vi "OverlayTest.vi"() -> ()   [LabVIEW 2015]
panel:
  in  "Listbox":i32(listbox)
  out "Center":dbl
  in  "BullseyeLocation":T1={"X Center"=364, "Y Center"=60, "Height"=92, "Width"=57}
  out "Image":T2(plugin-control)
  in  "index":i32
  out "Object Info.Bounding Box":T3={"X Left"=341, "Y Top"=61, "X Right"=396, "Y Bottom"=95}
  in  "End Point 2":cluster{"X":i32, "Y":i32}={"X"=450, "Y"=320}
  in  "Start Point 2":cluster{"X":i32, "Y":i32}={"X"=600, "Y"=480}
  in  "End Point":cluster{"X":i32, "Y":i32}={"X"=160, "Y"=320}
  in  "Start Point":cluster{"X":i32, "Y":i32}={"X"=15, "Y"=480}
  in  "stop":bool
  out "Masked":T2(plugin-control)
  out "Box Center":dbl=367.3384704589844
  in  "BallPresent":T4={"X Offset"=140, "Y Offset"=0, "Diameter"=20}
  in  "FixedMarkers":dbl[](array[numeric])
  in  "Value":dbl(slide)=1.0 scale=0.0..1.0
  in  "LinearLocation":T5={"X Offset"=10, "Y Offset"=170, "Height"=300, "Width"=10}
  in  "Values":dbl[](array[numeric])=[5000.0, 5129.0, 6.2, 1568.0]
  in  "Headers":string[](array[string])=["RPM:  ", "RPMt: ", "Box Pos: ", "Blah: "]
  in  "Present?":bool
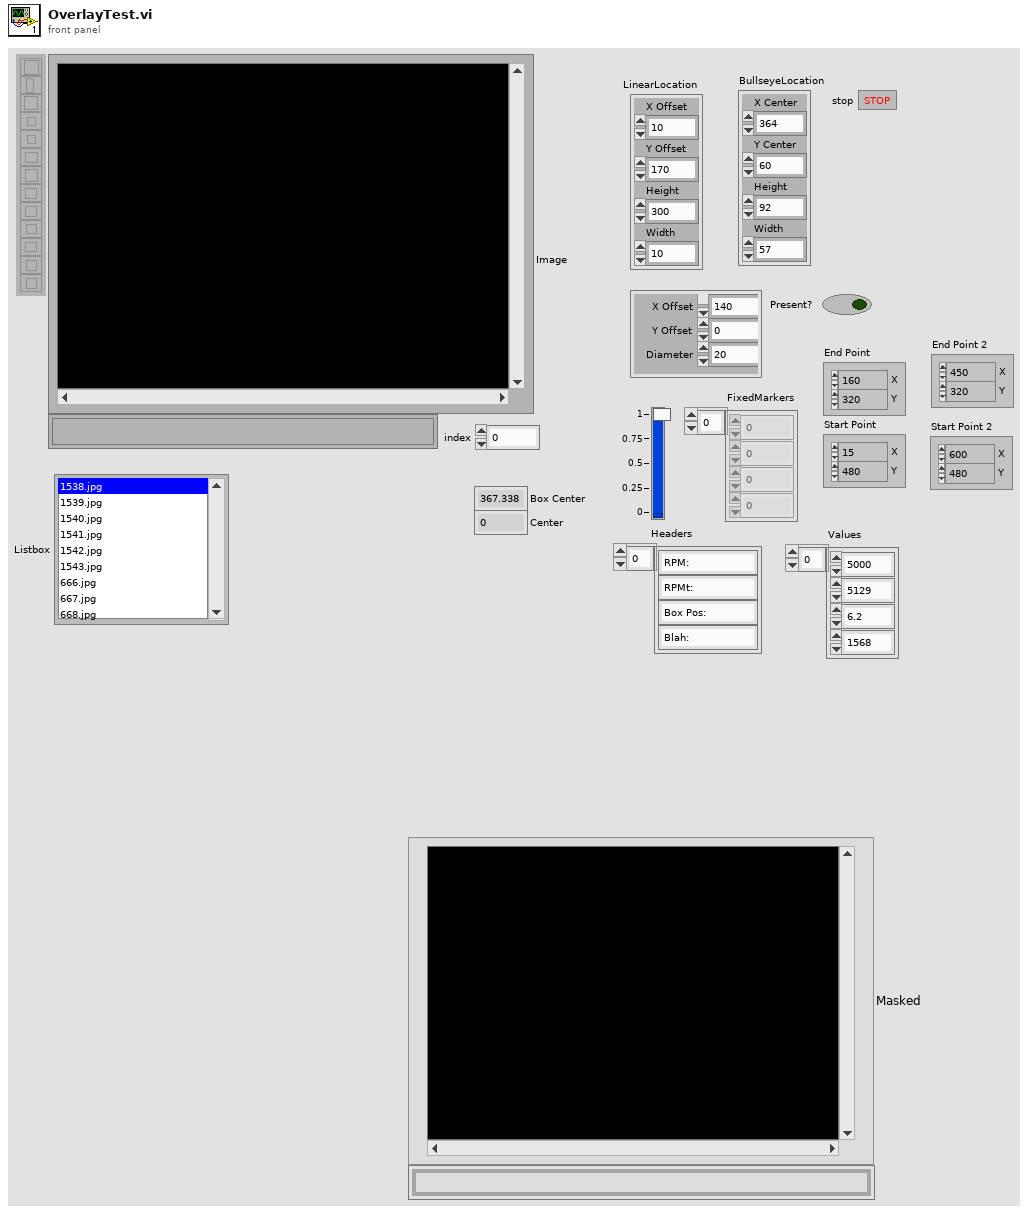
[diagram p1: front panel]
types:
  T1 = cluster{"X Center":i32, "Y Center":i32, "Height":i32, "Width":i32}
  T2 = typedef "IMAQ Image.ctl" = refnum<image>
  T3 = cluster{"X Left":i32, "Y Top":i32, "X Right":i32, "Y Bottom":i32}
  T4 = cluster{"X Offset":i32, "Y Offset":i32, "Diameter":i32}
  T5 = cluster{"X Offset":i32, "Y Offset":i32, "Height":i32, "Width":i32}
  T6 = typedef "Image Type" = u32
  T7 = cluster{"Area":sgl, "Object Info":cluster{"Object Center":cluster{"X":sgl, "Y":sgl}, "Bounding Box":cluster{"X Left":i32, "Y Top":i32, "X Right":i32, "Y Bottom":i32}, "Area":sgl, "Orientation":sgl, "Aspect Ratio":sgl, "Nb Holes":i32}}[]
  T8 = typedef "Scores.ctl" = cluster{"Bounding box":cluster{"left":dbl, "top":dbl, "right":dbl, "bottom":dbl}, "Aspect Ratio":dbl, "Area to CH":dbl, "X Mask":dbl, "Y Mask":dbl, "Moment":dbl, "Center":dbl}
  T9 = cluster{cluster{"Left":dbl, "Top":dbl, "Right":dbl, "Bottom":dbl}, "Scores":dbl[], cluster{"Long":dbl, "Short":dbl}}[]
  T10 = cluster{cluster{"Left":dbl, "Top":dbl, "Right":dbl, "Bottom":dbl}, "Scores":dbl[], cluster{"Long":dbl, "Short":dbl}}
  T11 = cluster{"Area":sgl, "Object Info":cluster{"Object Center":cluster{"X":sgl, "Y":sgl}, "Bounding Box":cluster{"X Left":i32, "Y Top":i32, "X Right":i32, "Y Bottom":i32}, "Area":sgl, "Orientation":sgl, "Aspect Ratio":sgl, "Nb Holes":i32}}
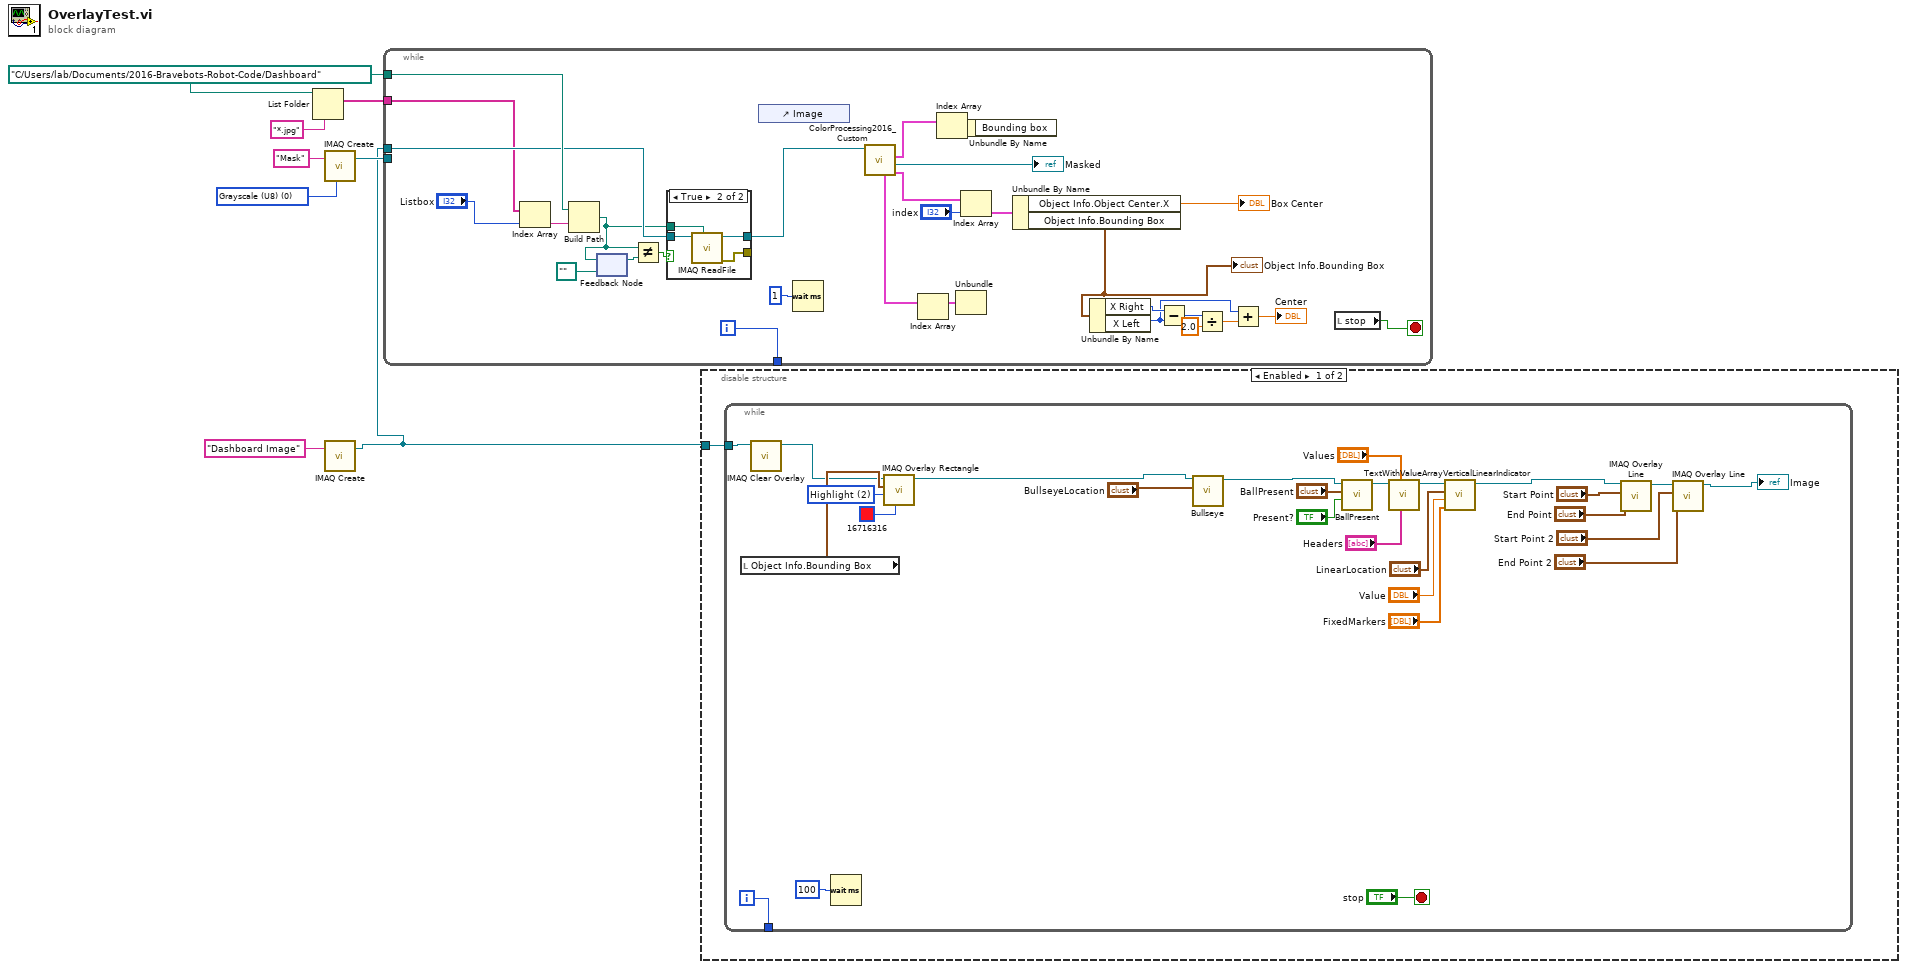
[diagram p0: block diagram]
diagram:
  w3 = path "C:/Users/lab/Documents/2016-Bravebots-Robot-Code/Dashboard" ("File Path")
  w7 = T6 0 items=["Grayscale (U8)", "Grayscale (I16)", "Grayscale (SGL)", "Complex (CSG)", "RGB (U32)", "HSL (U32)", "RGB (U64)", "Grayscale (U16)"] ("Image Type")
  n1 = List Folder(path=w3, pattern="*.jpg") -> (filenames=w2:string[])  [unwired: 2 in, 3 out]
  n2 = call "IMAQ Create"("Image Name"="Mask", "Image Type"=w7) -> ("New Image"=w5:T2)  [unwired: 2 in, 2 out]
  n3 = call "IMAQ Create"("Image Name"="Dashboard Image") -> ("New Image"=w1:T2)  [unwired: 3 in, 2 out]
  n4 = while {
    tunnel: w1 -> [w14]
    tunnel: w5 -> [_]
    tunnel: [w32] -> _
    tunnel: w3 -> [w18]
    tunnel: w2 -> [w12]
    i -> [w32]
    stop <- w31 stop-if-true
    n5 = Index Array(array=w12, index="Listbox") -> (element=w10:string)
    n6 = Build Path(base path=w18, name or relative path=w10) -> (appended path=w9:path)
    n7 = feedback #1(path "" ("appended path")) -> (w17:path)
    n8 = feedback-in #1(w9) -> ()
    n9 = Not Equal?(x=w9, y=w17) -> (x != y?=w15:bool)
    n10 = case shown="True" w15 {
      tunnel: [w38 w42] -> w13
      tunnel: [_ w41] -> _
      tunnel: w14 -> [w38 w40]
      tunnel: w9 -> [_ w39]
      frame False {
      }
      frame True {
        n11 = call "IMAQ ReadFile"("File Path"=w39, "Image"=w40) -> ("error out"=w41:errorcluster, "Image Out"=w42:T2)  [unwired: 5 in, 3 out]
      }
    }
    n12 = control-ref of="Image"() -> ()  [unwired: 1 out]
    n13 = Wait (ms)(milliseconds to wait=u32 1) -> ()  [unwired: 1 out]
    n14 = call "ColorProcessing2016_Custom.vi"("Original"=w13) -> ("Blob array"=w35:T7, "Masked"=→"Masked":T2, "Targets"=w21:T8[], "Scored Particle Info 2"=w29:T9)  [unwired: 6 in, 1 out]
    n15 = Index Array(array=w29) -> (element=w28:T10)  [unwired: 1 in]
    n16 = Index Array(array=w21) -> (element=w20:T8)  [unwired: 1 in]
    n17 = Unbundle(w28) -> ()  [unwired: 3 out]
    n18 = Unbundle By Name(w20) -> ()  [unwired: 1 out]
    n19 = Index Array(array=w35, index="index") -> (element=w36:T11)
    n20 = Unbundle By Name(w36) -> ("Object Info.Object Center.X"=→"Box Center":sgl, "Object Info.Bounding Box"=w19:T3)
    "Object Info.Bounding Box" <- w19
    n21 = Unbundle By Name(w19) -> ("X Right"=w24:i32, "X Left"=w22:i32)
    n22 = Subtract(x=w24, y=w22) -> (x-y=w27:i32)
    n23 = Divide(x=w27, y=2.0) -> (x/y=w25:dbl)
    n24 = Add(x=w22, y=w25) -> (x+y=→"Center":dbl)
    n25 = local read "stop"() -> (w31:bool)
  }
  n26 = disable-structure shown="Enabled" {
    disable-tunnel: w1 -> [w43 _]
    frame Enabled {
      n27 = while {
        tunnel: w43 -> [w70]
        tunnel: [w60] -> _
        i -> [w60]
        stop <- "stop" stop-if-true
        w50 = u32 2 items=["Frame", "Fill", "Highlight"] ("Drawing Mode (Frame)")
        n28 = local read "Object Info.Bounding Box"() -> (w48:T3)
        n29 = call "IMAQ Clear Overlay"("Image"=w70) -> ("Image Out"=w47:T2)  [unwired: 9 in, 1 out]
        n30 = Wait (ms)(milliseconds to wait=u32 100) -> ()  [unwired: 1 out]
        n31 = call "IMAQ Overlay Rectangle"("Color"=u32 16716316, "Drawing Mode (Frame)"=w50, "Rectangle"=w48, "Image"=w47) -> ("Image Out"=w46:T2)  [unwired: 6 in, 1 out]
        n32 = call "Bullseye.vi"("SizeAndLocation"="BullseyeLocation", "Image in"=w46) -> ("Image out"=w68:T2)  [unwired: 9 in]
        n33 = call "BallPresent.vi"("Present?"="Present?", "SizeAndLocation"="BallPresent", "Image in"=w68) -> ("Image out"=w65:T2)  [unwired: 8 in]
        n34 = call "TextWithValueArray.vi"("Headers"="Headers", "Values"="Values", "Image in"=w65) -> ("Image out"=w64:T2)  [unwired: 8 in]
        n35 = call "VerticalLinearIndicator.vi"("FixedMarkers"="FixedMarkers", "Value"="Value", "SizeAndLocation"="LinearLocation", "Refnum in"=w64) -> ("Refnum out"=w56:T2)  [unwired: 7 in]
        n36 = call "IMAQ Overlay Line"("End Point"="End Point", "Start Point"="Start Point", "Image"=w56) -> ("Image Out"=w53:T2)  [unwired: 7 in, 1 out]
        n37 = call "IMAQ Overlay Line"("End Point"="End Point 2", "Start Point"="Start Point 2", "Image"=w53) -> ("Image Out"=→"Image":T2)  [unwired: 7 in, 1 out]
      }
    }
    frame Disabled {
    }
  }
